vi "CalibrationtoXML.vi"(1 "Calibrations":T1=[{"Gain"=0.0, "Offset (V)"=0.0, "Name"=""}] {"Offset (V)" format="%_6p"; "Gain" format="%_6p"}, 2 "XML File Path":path) -> (0 "MD5 message-digest":string)   [LabVIEW 2018]
uses:
  Calibrations.ctl
  <vilib>/Utility/xml.llb/Write to XML File(string).vi
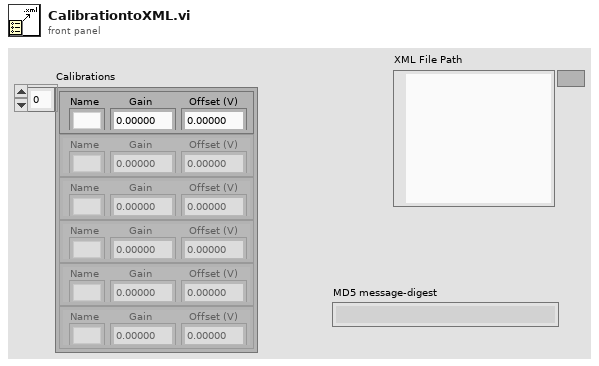
[diagram p1: front panel]
types:
  T1 = typedef "Calibrations.ctl" = cluster{"Gain":dbl, "Offset (V)":dbl, "Name":string}[]
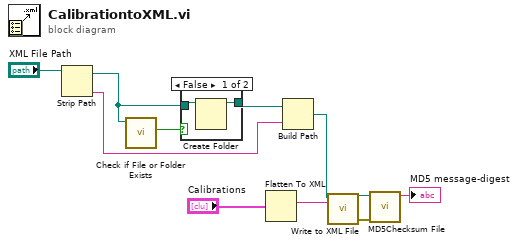
[diagram p0: block diagram]
diagram:
  n1 = Strip Path(path="XML File Path") -> (stripped path=w9:path, name=w7:string)
  n2 = call <vilib>:"Check if File or Folder Exists.vi"("path"=w9) -> ("file or folder exists?"=w10:bool)  [unwired: 8 in, 2 out]
  n3 = case shown="False" w10 {
    tunnel: w9 -> [w13 w14]
    tunnel: [w12 w14] -> w8
    frame False {
      n4 = Create Folder(path (use dialog)=w13) -> (created path=w12:path)  [unwired: 2 in, 2 out]
    }
    frame True {
    }
  }
  n5 = Flatten To XML(anything="Calibrations") -> (xml string=w11:string)
  n6 = Build Path(base path=w8, name or relative path=w7) -> (appended path=w6:path)
  n7 = call-poly <vilib>:"Write to XML File.vi"("XML Input"=w11, "XML File Path"=w6) -> ("error out"=w2:errorcluster, "XML File Path(duplicate)"=w1:path)  [unwired: 7 in, 1 out]
  n8 = call <vilib>:"MD5Checksum File.vi"("error in (no error)"=w2, "Path"=w1) -> ("MD5 message-digest"=→"MD5 message-digest":string)  [unwired: 8 in, 1 out]
